vi "LM 2D Gaussian ACF + Flow and gradient (Global).vi"(3 "output control":T1, 4 "data":variant, 5 "X":dbl[](array[numeric]), 6 "a":dbl[](array[numeric])) -> (0 "error out":errorcluster, 1 "f'(X,a)":dbl[][](array[numeric]), 2 "f(X,a)":dbl[](array[numeric]))   [LabVIEW 2021, in "Fits.lvlib"]
doc: "This template is the starting point for creating a model function to be passed to the Nonlinear Curve Fit.vi."
uses:
  <vilib>/gmath/NumericalOptimization/LM_output select.ctl
  Variant/Variant to Data/Variant to I32.vi
  Fits.lvlib
  Variant/Variant to Data/Variant to Data.lvlib
  <vilib>/gmath/NI_Gmath.lvlib
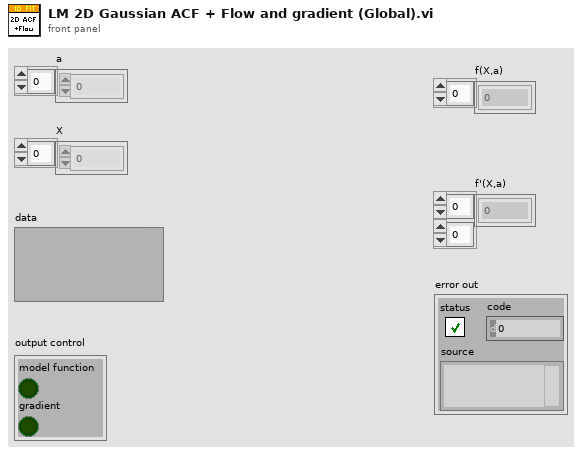
[diagram p1: front panel]
types:
  T1 = typedef "NI_Gmath.lvlib/LM_output select.ctl" = cluster{"model function":bool, "gradient":bool}
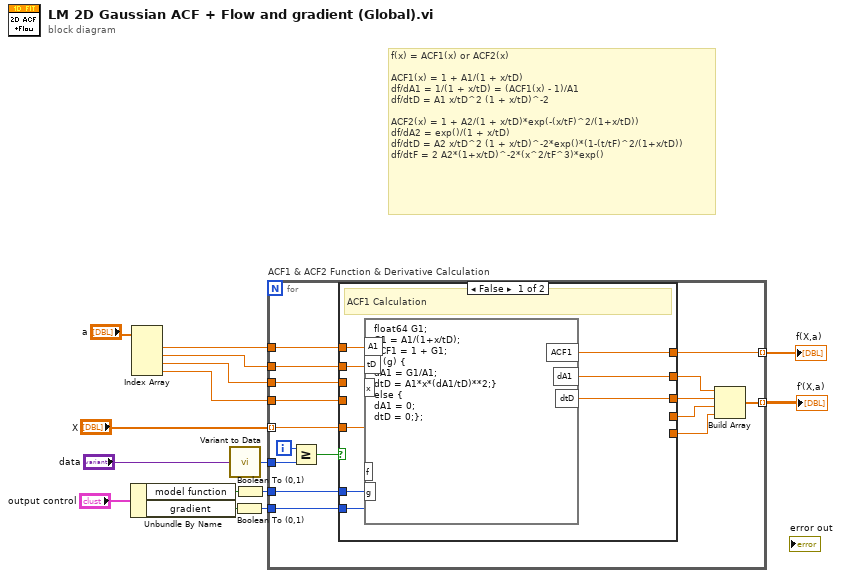
[diagram p0: block diagram]
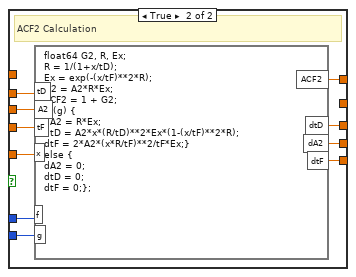
[diagram p2: hidden frame]
diagram:
  # "f(x) = ACF1(x) or ACF2(x)\n\nACF1(x) = 1 + A1/(1 + x/tD)\ndf/dA1 = 1/(1 + x/tD) = (ACF1(x) - 1)/A1\ndf/dtD = A1 x/tD^2 (1 + x/tD)^-2\n\nACF2(x) = 1 + A2/(1 + x/tD)*exp(-(x/tF)^2/(1+x/tD))\ndf/dA2 = exp()/(1 + x/tD)\ndf/dtD = A2 x/tD^2 (1 + x/tD)^-2*exp()*(1-(t/tF)^2/(1+x/tD))\ndf/dtF = 2 A2*(1+x/tD)^-2*(x^2/tF^3)*exp()"
  n1 = Unbundle By Name("output control") -> ("model function"=w6:bool, "gradient"=w4:bool)
  n2 = Index Array(array="a") -> (element #1=w12:dbl, element #2=w11:dbl, element #3=w2:dbl, element #4=w1:dbl)  [unwired: 4 in]
  n3 = call-poly "Variant to Data.vi"("Variant"="data") -> ("Value"=w9:i32)  [unwired: 8 in]
  n4 = Boolean To (0,1)(Boolean=w4) -> (0, 1=w3:i16)
  n5 = Boolean To (0,1)(Boolean=w6) -> (0, 1=w5:i16)
  n6 = for "ACF1 & ACF2 Function & Derivative Calculation" {
    tunnel: "X" -> [w29] mode=indexing
    tunnel: w12 -> [w31]
    tunnel: w11 -> [w30]
    tunnel: w9 -> [w27]
    tunnel: [w25] -> w8 mode=indexing
    tunnel: [w22] -> w7 mode=indexing
    tunnel: w5 -> [w21]
    tunnel: w3 -> [w20]
    tunnel: w2 -> [w19]
    tunnel: w1 -> [w18]
    i -> [w28]
    n7 = Greater Or Equal?(x=w28, y=w27) -> (x >= y?=w26:bool)
    n8 = case shown="False" w26 {
      tunnel: w31 -> [w39 _]
      tunnel: w30 -> [w38 w49]
      tunnel: w29 -> [w37 w48]
      tunnel: [w36 w47] -> w25
      tunnel: [w35 _] -> w24
      tunnel: [w34 w46] -> w23
      tunnel: w21 -> [w33 w45]
      tunnel: w20 -> [w32 w44]
      tunnel: w19 -> [_ w43]
      tunnel: w18 -> [_ w42]
      tunnel: [_ w41] -> w17
      tunnel: [_ w40] -> w16
      frame False {
        # "ACF1 Calculation"
        n9 = formula code="float64 G1;\nG1 = A1/(1+x/tD);\nACF1 = 1 + G1;\nif (g) {\ndA1 = G1/A1;\ndtD = A1*x*(dA1/tD)**2;}\nelse {\ndA1 = 0;\ndtD = 0;};"("A1"=w39, "tD"=w38, "x"=w37, "f"=w33, "g"=w32) -> ("dA1"=w35:dbl, "dtD"=w34:dbl, "ACF1"=w36:dbl)
      }
      frame True {
        # "ACF2 Calculation"
        n10 = formula code="float64 G2, R, Ex;\nR = 1/(1+x/tD);\nEx = exp(-(x/tF)**2*R);\nG2 = A2*R*Ex;\nACF2 = 1 + G2;\nif (g) {\ndA2 = R*Ex;\ndtD = A2*x*(R/tD)**2*Ex*(1-(x/tF)**2*R);\ndtF = 2*A2*(x*R/tF)**2/tF*Ex;}\nelse {\ndA2 = 0;\ndtD = 0;\ndtF = 0;};"("tD"=w49, "x"=w48, "f"=w45, "g"=w44, "A2"=w43, "tF"=w42) -> ("dA2"=w41:dbl, "dtD"=w46:dbl, "ACF2"=w47:dbl, "dtF"=w40:dbl)
      }
    }
    n11 = Build Array(w24, w23, w17, w16) -> (w22:dbl[])
  }
  "f(X,a)" <- w8
  "f'(X,a)" <- w7
